vi "usbPIP.vi"(8 "error in (no error)":errorcluster) -> (0 "error out":errorcluster, 2 "Boolean":bool, 3 "USB-16":string)   [LabVIEW 2018]
uses:
  Global_1259.vi
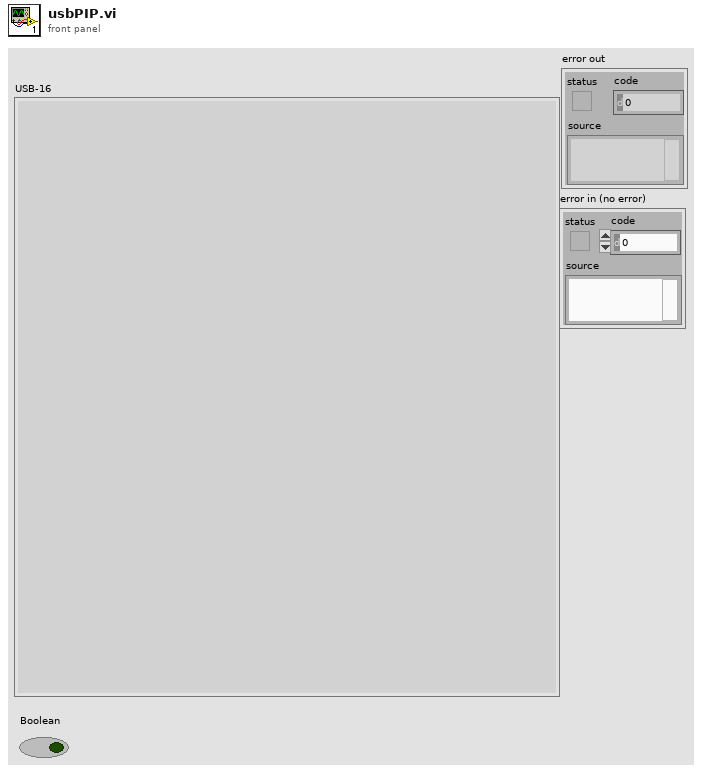
[diagram p1: front panel]
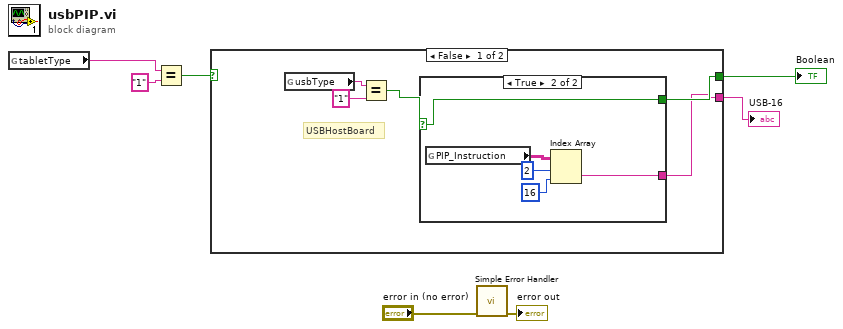
[diagram p0: block diagram]
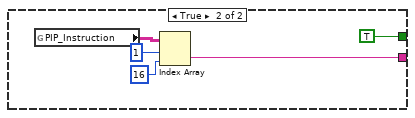
[diagram p3: hidden frame]
diagram:
  n1 = global read "Global_1259.vi" "tabletType"() -> (w6:string)
  n2 = Equal?(x=w6, y="1") -> (x = y?=w4:bool)
  n3 = case shown="False" w4 {
    tunnel: [w9 TRUE] -> w5
    tunnel: [w8 w19] -> w7
    frame False {
      # "USBHostBoard"
      n4 = global read "Global_1259.vi" "usbType"() -> (w12:string)
      n5 = Equal?(x=w12, y="1") -> (x = y?=w10:bool)
      n6 = case shown="True" w10 {
        selector: w10 -> [w13 w15]
        tunnel: [w13 w15] -> w9
        tunnel: [_ w14] -> w8
        frame False {
        }
        frame True {
          n7 = global read "Global_1259.vi" "PIP_Instruction"() -> (w18:string[][])
          n8 = Index Array(array=w18, index (row)=2 ("disabled index (row)"), index (col)=16 ("disabled index (col)")) -> (element=w14:string)
        }
      }
    }
    frame True {
      n9 = global read "Global_1259.vi" "PIP_Instruction"() -> (w22:string[][])
      n10 = Index Array(array=w22, index (row)=1 ("disabled index (row)"), index (col)=16 ("disabled index (col)")) -> (element=w19:string)
    }
  }
  "USB-16" <- w7
  "Boolean" <- w5
  n11 = call <vilib>:"Simple Error Handler.vi"("error in (no error)"="error in (no error)") -> ("error out"=→"error out":errorcluster)  [unwired: 4 in, 4 out]
